vi "Determine Warnings.vi"(8 "error in (no error)":errorcluster, 9 "Min Temp":dbl, 10 "Max Temp":dbl, 11 "Current Temp":dbl) -> (0 "error out":errorcluster, 1 "Warning?":bool, 2 "Warning Text":string)   [LabVIEW 2010]
doc: "This is a solution VI in the LabVIEW Core I course. In this exercise, you use the error in cluster to abort execution of the VI."
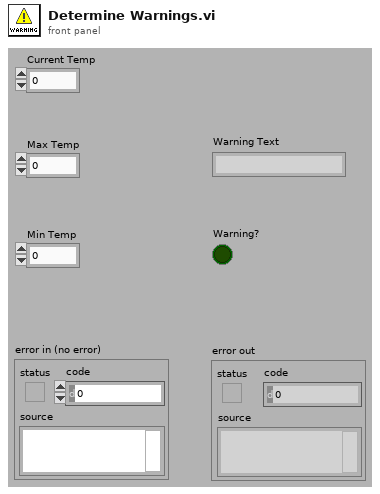
[diagram p1: front panel]
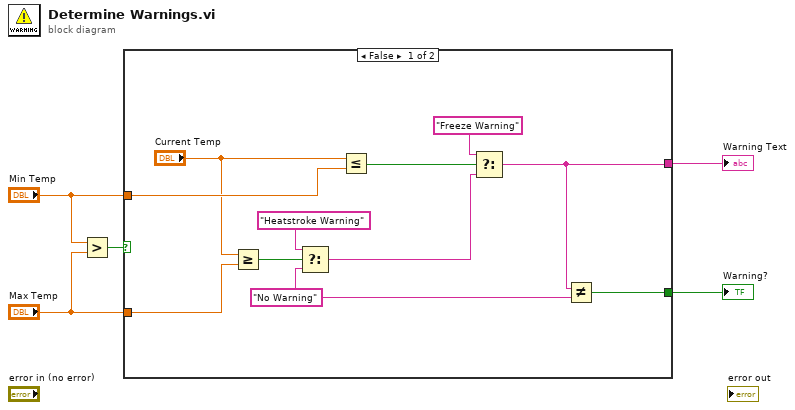
[diagram p0: block diagram]
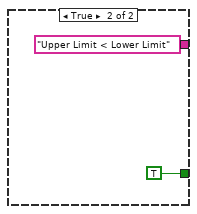
[diagram p2: hidden frame]
diagram:
  n1 = Greater?(x="Min Temp", y="Max Temp") -> (0:w3:bool)
  n2 = case shown="False" w3 {
    tunnel: [w16 "Upper Limit < Lower Limit" ("f")] -> w5
    tunnel: [w15 TRUE] -> w4
    tunnel: "Max Temp" -> [w14 _]
    tunnel: "Min Temp" -> [w11 _]
    frame False {
      w6 = "No Warning" ("f")
      n3 = Greater Or Equal?(x="Current Temp", y=w14) -> (x >= y?=w13:bool)
      n4 = Select(t="Heatstroke Warning", s=w13, f=w6) -> (s? t:f=w7:string)
      n5 = Less Or Equal?(x="Current Temp", y=w11) -> (x <= y?=w8:bool)
      n6 = Select(t="Freeze Warning", s=w8, f=w7) -> (s? t:f=w16:string)
      n7 = Not Equal?(x=w16, y=w6) -> (x != y?=w15:bool)
    }
    frame True {
    }
  }
  "Warning Text" <- w5
  "Warning?" <- w4
